vi "Engine Offset (Transfer).vi"(8 "error in (no error)":errorcluster, 11 "Transfer Configuration in":T1 {"channel configurations"."buffer offset" format="%d bytes"}) -> (0 "error out":errorcluster, 2 "engine offset":u64, 3 "Transfer Configuration out":T1 {"channel configurations"."buffer offset" format="%d bytes"})   [LabVIEW 2017, in "DSF Core.lvlib"]
uses:
  DSF Core.lvlib
  Controls/DSF Engine Transfer Configuration.ctl
  Controls/DSF Byte Order.ctl
  Controls/DSF Engine Channel Configuration.ctl
  Controls/DSF Data Type.ctl
  Controls/DSF Settings Info.ctl
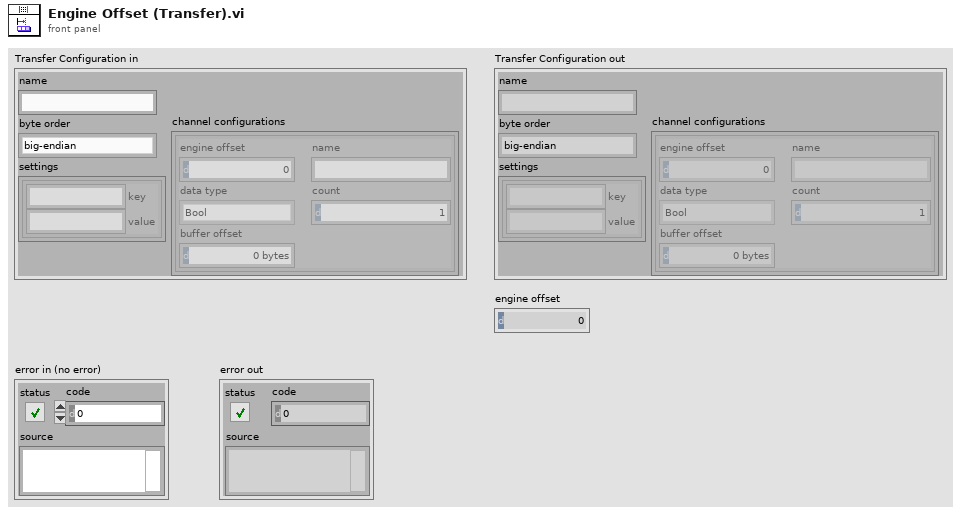
[diagram p1: front panel]
types:
  T1 = typedef "DSF Core.lvlib/DSF Engine Transfer Configuration.ctl" = cluster{"name":string, "byte order":T2, "channel configurations":T3[], "settings":T5}
  T2 = typedef "DSF Core.lvlib/DSF Byte Order.ctl" = enum8{"big-endian", "little-endian"}
  T3 = typedef "DSF Core.lvlib/DSF Engine Channel Configuration.ctl" = cluster{"engine offset":u64, "name":string, "data type":T4, "count":u64, "buffer offset":u64}
  T4 = typedef "DSF Core.lvlib/DSF Data Type.ctl" = enum8{"Bool", "SGL", "DBL", "I8", "I16", "I32", "I64", "U8", "U16", "U32", "U64"}
  T5 = typedef "DSF Core.lvlib/DSF Settings Info.ctl" = cluster{"key":string, "value":string}[]
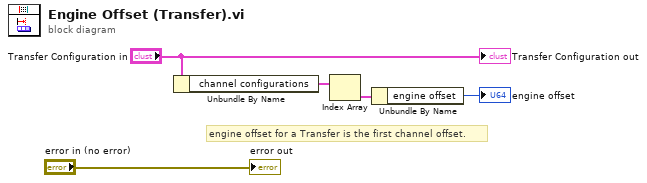
[diagram p0: block diagram]
diagram:
  # "engine offset for a Transfer is the first channel offset."
  n1 = Unbundle By Name("Transfer Configuration in") -> ("channel configurations"=w4:T3[])
  n2 = Index Array(array=w4) -> (element=w3:T3)  [unwired: 1 in]
  n3 = Unbundle By Name(w3) -> ("engine offset"=→"engine offset":u64)
  "Transfer Configuration out" <- "Transfer Configuration in"
  "error out" <- "error in (no error)"
